vi "Stop.vi"(8 "error in (no error)":errorcluster, 9 "timeout in ms (-1)":i32=-1, 11 "Execution UI In":refnum<class "Execution UI V2.lvclass">) -> (0 "error out":errorcluster, 1 "timed out?":bool, 3 "Execution UI Out":refnum<class "Execution UI V2.lvclass">)   [LabVIEW 2020, in "Execution UI V2.lvclass"]
uses:
  Execution UI V2.lvclass
  C:/Git/astemes-lunit/source/Application Framework/Process Classes/Process/Process.lvclass
  Application Framework/Process Classes/Process/Process.lvclass/Process.ctl
  Execution UI V2.lvclass/Execution UI V2.ctl
  Application Framework/Process Classes/Process/Process.lvclass
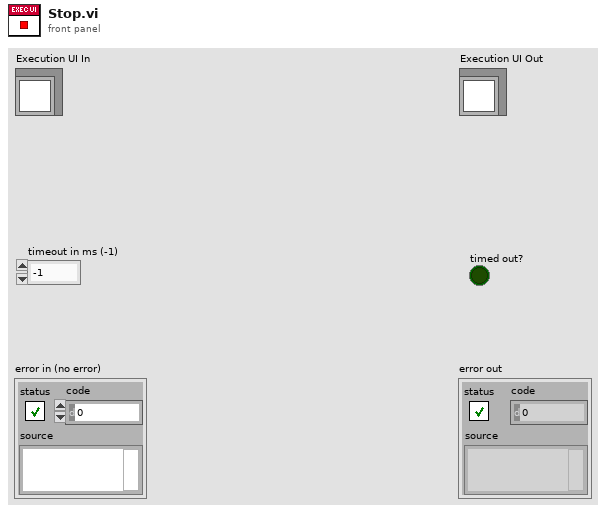
[diagram p1: front panel]
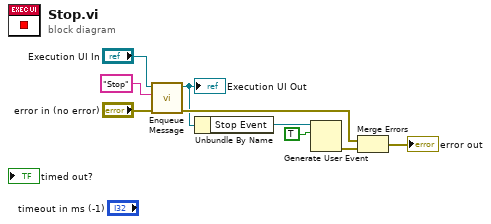
[diagram p0: block diagram]
diagram:
  n1 = call "Enqueue Message.vi"("error in (no error)"="error in (no error)", "Message"="Stop", "Process In"="Execution UI In") -> ("error out"=w4:errorcluster, "Process Out"=w2:refnum<class "Execution UI V2.lvclass">)  [unwired: 7 in]
  "Execution UI Out" <- w2
  n2 = Unbundle By Name(w2) -> ("Stop Event"=w8:refnum<user-event>)
  n3 = Generate User Event(user event=w8, event data cluster=TRUE ("event data")) -> (error out=w5:errorcluster)  [unwired: 2 in, 1 out]
  n4 = Merge Errors(w4, w5) -> (→"error out":errorcluster)
